vi "queue_Close_Test.vi"() -> ()   [LabVIEW 2018]
uses:
  Controls/Enums/AO_Loop_Enum.ctl
panel:
  out "Write":i32
  out "init":i32
  in  "Send":bool
  in  "error 2":errorcluster
  out "error out":errorcluster
  in  "error":errorcluster
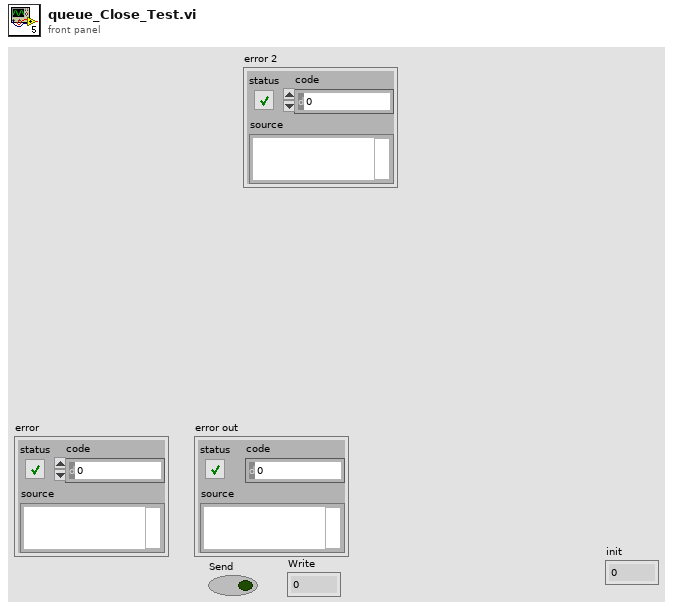
[diagram p1: front panel]
types:
  T1 = typedef "AO_Loop_Enum.ctl" = enum16{"AO_Init", "AO_Write", "AO_Exit"}
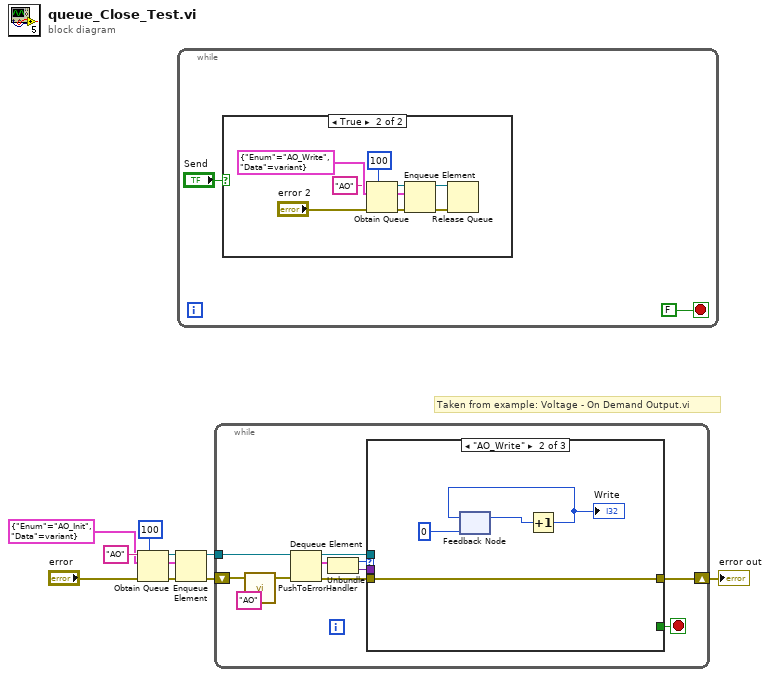
[diagram p0: block diagram]
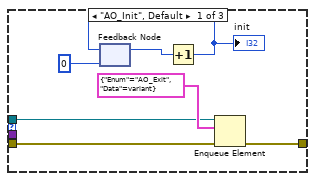
[diagram p3: hidden frame]
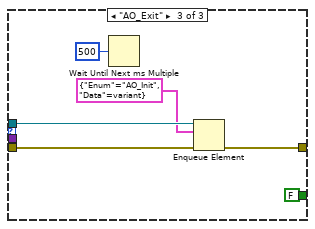
[diagram p4: hidden frame]
diagram:
  w5 = cluster{"Enum":T1, "Data":variant} {"Enum"=enum."AO_Init", "Data"=variant}
  # "Taken from example: Voltage - On Demand Output.vi"
  n1 = Obtain Queue(max queue size (-1, unlimited)=100, name (unnamed)="AO", element data type=w5, error in (no error)="error") -> (queue out=w9:refnum<queue>, error out=w7:errorcluster)  [unwired: 1 in, 1 out]
  n2 = Enqueue Element(queue=w9, element=w5, error in (no error)=w7) -> (queue out=w8:refnum<queue>, error out=w1:errorcluster)  [unwired: 1 in, 1 out]
  n3 = while {
    stop <- FALSE stop-if-true
    n4 = case shown="True" "Send" {
      frame False {
      }
      frame True {
        w17 = cluster{"Enum":T1, "Data":variant} {"Enum"=enum."AO_Write", "Data"=variant}
        n5 = Obtain Queue(max queue size (-1, unlimited)=100, name (unnamed)="AO", element data type=w17, error in (no error)="error 2") -> (queue out=w14:refnum<queue>, error out=w15:errorcluster)  [unwired: 1 in, 1 out]
        n6 = Enqueue Element(queue=w14, element=w17, error in (no error)=w15) -> (queue out=w12:refnum<queue>, error out=w13:errorcluster)  [unwired: 1 in, 1 out]
        n7 = Release Queue(queue=w12, error in (no error)=w13) -> ()  [unwired: 1 in, 3 out]
      }
    }
  }
  n8 = while {
    tunnel: w8 -> [w28]
    shift-right: [w30] -> w3
    shift-left: w1 -> [w21]
    stop <- w23 stop-if-true
    n9 = call "PushToErrorHandler.vi"("ErrorIn"=w21, "ErrorLocation"="AO") -> ("ErrorOut"=w22:errorcluster)  [unwired: 5 in]
    n10 = Dequeue Element(queue=w28, error in (no error)=w22) -> (queue out=w24:refnum<queue>, element=w27:cluster{"Enum":T1, "Data":variant}, error out=w29:errorcluster)  [unwired: 1 in, 1 out]
    n11 = Unbundle(w27) -> ("Enum"=w26:T1, "Data"=w25:variant)
    n12 = case shown="\"AO_Write\"" w26 {
      tunnel: w29 -> [w33 w41 w46]
      tunnel: [w32 w41 w45] -> w30
      tunnel: w25 -> [_ _ _]
      tunnel: w24 -> [w31 _ w44]
      tunnel: [_ _ FALSE] -> w23
      frame "AO_Init", Default {
        n13 = feedback #1(0) -> (w36:i32)
        n14 = Increment(x=w36) -> (x+1=w35:i32)
        "init" <- w35
        n15 = feedback-in #1(w35) -> ()
        n16 = Enqueue Element(queue=w31, element=cluster{"Enum":T1, "Data":variant} {"Enum"=enum."AO_Exit", "Data"=variant}, error in (no error)=w33) -> (error out=w32:errorcluster)  [unwired: 1 in, 2 out]
      }
      frame "AO_Write" {
        n17 = feedback #2(0) -> (w39:i32)
        n18 = Increment(x=w39) -> (x+1=w38:i32)
        "Write" <- w38
        n19 = feedback-in #2(w38) -> ()
      }
      frame "AO_Exit" {
        n20 = Wait Until Next ms Multiple(millisecond multiple=u32 500) -> ()  [unwired: 1 out]
        n21 = Enqueue Element(queue=w44, element=cluster{"Enum":T1, "Data":variant} {"Enum"=enum."AO_Init", "Data"=variant}, error in (no error)=w46) -> (error out=w45:errorcluster)  [unwired: 1 in, 2 out]
      }
    }
  }
  "error out" <- w3
